vi "Process_LockRef.vi"(0 "ref in":T2, 3 "error in":errorcluster) -> (6 "ref out":T2, 7 "Lock ref out":T1, 9 "error out":errorcluster)   [LabVIEW 2015]
panel:
  out "Timed out":bool
  in  "ms timeout (-1)":i32=-1
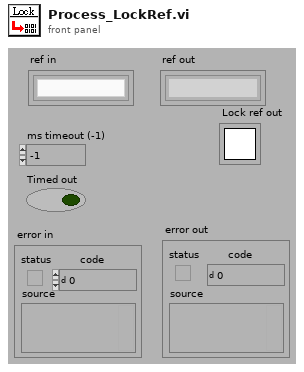
[diagram p1: front panel]
types:
  T1 = typedef "Semaphore RefNum" = refnum<k1>
  T2 = typedef "Error站_ref.ctl" = refnum<k1>
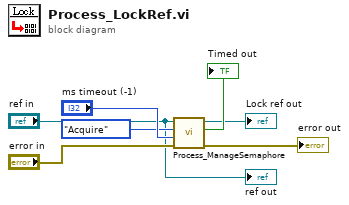
[diagram p0: block diagram]
diagram:
  n1 = call "Process_ManageSemaphore.vi"("error in (no error)"="error in", "ms timeout (-1)"="ms timeout (-1)", "Method (Acquire)"=enum8{"Acquire", "Destroy"}."Acquire", "ref"="ref in") -> ("error out"=→"error out":errorcluster, "Timed out"=→"Timed out":bool, "semaphore out"=→"Lock ref out":T1)  [unwired: 1 in]
  "ref out" <- "ref in"
